vi "Get Running.vi"(8 "error in (no error)":errorcluster, 11 "ArrayManager in":refnum<class "ArrayManager.lvclass">) -> (0 "error out":errorcluster, 2 "Running":bool, 3 "ArrayManager out":refnum<class "ArrayManager.lvclass">)   [LabVIEW 2020, in "OOPanel.lvlib" / "ArrayManager.lvclass"]
uses:
  ArrayManager.lvclass
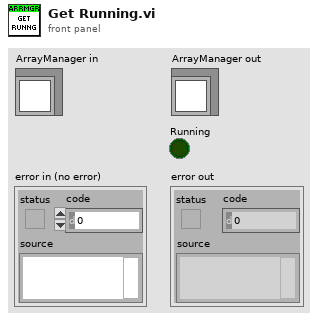
[diagram p1: front panel]
types:
  T1 = typedef "OOPanel.lvlib/ArrayManager.lvclass/State Ref.ctl" = cluster{"Running":bool, "Borders":bool, "Total Height":dbl, "Scroll Visible":bool, "Background":u32}
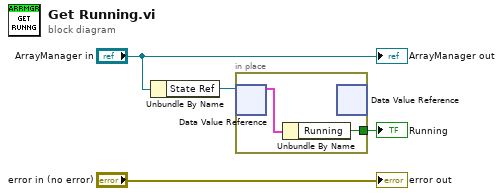
[diagram p0: block diagram]
diagram:
  n1 = Unbundle By Name("ArrayManager in") -> ("State Ref"=w3:refnum<data-value>)
  n2 = in-place {
    in-place-border: [w5] -> w1
    n3 = in-place-dvr #1(w3) -> (w6:T1)  [unwired: 1 out]
    n4 = Unbundle By Name(w6) -> ("Running"=w5:bool)
    n5 = in-place-dvr #1() -> ()  [unwired: 1 in, 2 out]
  }
  "Running" <- w1
  "error out" <- "error in (no error)"
  "ArrayManager out" <- "ArrayManager in"
